vi "Set Mode.vi"(8 "error in (no error)":errorcluster, 10 "Mode":T1, 11 "Endpoint in":refnum<class "Endpoint.lvclass">) -> (0 "error out":errorcluster, 3 "Endpoint out":refnum<class "Endpoint.lvclass">)   [LabVIEW 2020, in "Stream.lvlib" / "Endpoint.lvclass"]
uses:
  Endpoint.lvclass
  Mode.ctl
  Endpoint.lvclass/Endpoint.ctl
  <vilib>/Utility/error.llb/Error Cluster From Error Code.vi
  <vilib>/ErrorRing/Error Ring.xnode
  Stream.lvlib
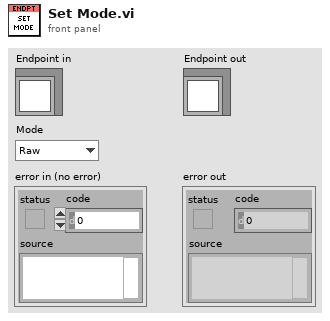
[diagram p1: front panel]
types:
  T1 = typedef "Stream.lvlib/Mode.ctl" = enum16{"Raw", "Buffered", "LineTerm", "Message"}
  T2 = typedef "Stream.lvlib/Endpoint.lvclass/Ref Data.ctl" = cluster{"URI":refnum<class "URI.lvclass">, "State Callbacks":T3[], "Open":bool, "Mode":T1, "Sniffer Callbacks":T3[]}
  T3 = typedef "Stream.lvlib/Endpoint.lvclass/State Callback.ctl" = cluster{"Owner":refnum<class>, "VI":refnum<vi>}
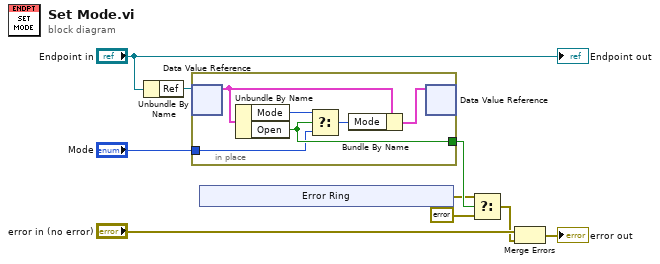
[diagram p0: block diagram]
diagram:
  n1 = Unbundle By Name("Endpoint in") -> ("Ref"=w8:refnum<data-value>)
  n2 = in-place {
    in-place-border: [w14] -> w6
    in-place-border: "Mode" -> [w13]
    n3 = in-place-dvr #1(w8) -> (w12:T2)  [unwired: 1 out]
    n4 = Unbundle By Name(w12) -> ("Mode"=w15:T1, "Open"=w14:bool)
    n5 = Select(t=w15, s=w14, f=w13) -> (s? t:f=w11:T1)
    n6 = Bundle By Name(cluster=w12, "Mode"=w11) -> (w10:T2)
    n7 = in-place-dvr #1(w10) -> ()  [unwired: 2 out]
  }
  n8 = xnode "Error Ring"() -> ("error out"=w5:errorcluster)
  n9 = Select(t=w5, s=w6, f=errorcluster {"status"=FALSE, "code"=0, "source"=""}) -> (s? t:f=w2:errorcluster)
  n10 = Merge Errors("error in (no error)", w2) -> (→"error out":errorcluster)
  "Endpoint out" <- "Endpoint in"
